vi "open.vi"(6 "error in (no error)":errorcluster, 9 "Device Index":u32) -> (0 "error out":errorcluster, 3 "DeviceRefnum Out":u64)   [LabVIEW 2015, in "rtlsdr.lvlib"]
doc: "RTLSDR_API int rtlsdr_open(rtlsdr_dev_t **dev, uint32_t index);"
uses:
  rtlsdr.lvlib
  rtlsdr/rtlsdr.dll
panel:
  in  "DeviceRefnum":u64
  out "function return":i32
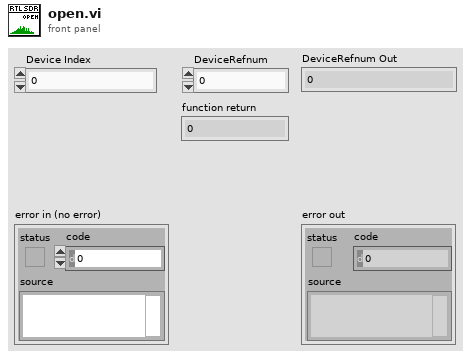
[diagram p1: front panel]
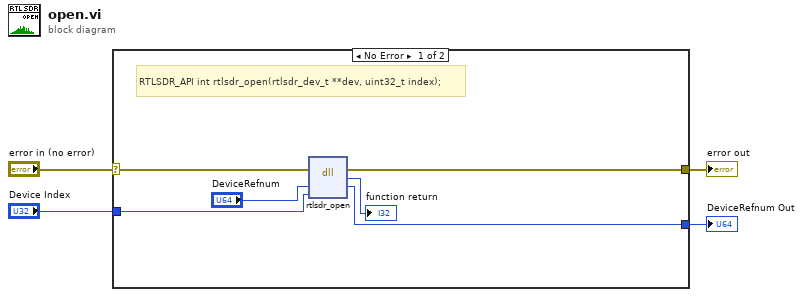
[diagram p0: block diagram]
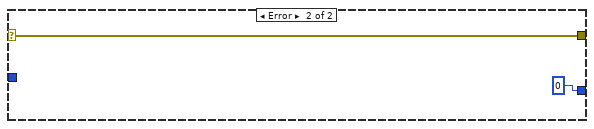
[diagram p2: hidden frame]
diagram:
  n1 = case shown="No Error" "error in (no error)" {
    selector: "error in (no error)" -> [w7 w12]
    tunnel: "Device Index" -> [w9 _]
    tunnel: [w5 w12] -> w3
    tunnel: [w8 u64 0 ("DeviceRefnum")] -> w2
    frame No Error {
      # "RTLSDR_API int rtlsdr_open(rtlsdr_dev_t **dev, uint32_t index);"
      n2 = dll-call lib="C:/Users/TheDoctor/Documents/Projects/Labview Libraries/rtlsdr/rtlsdr.*" fn="rtlsdr_open"(error in=w7, "DeviceRefnum"="DeviceRefnum", "index"=w9) -> (error out=w5:errorcluster, "return type"=→"function return":i32, "DeviceRefnum"=w8:u64)  [unwired: 3 in, 1 out]
    }
    frame Error {
    }
  }
  "error out" <- w3
  "DeviceRefnum Out" <- w2
